vi "MaskThreshold.vi"(7 "fraction":sgl=0.5, 10 "intervals":i32=30, 11 "Mean varS":sgl[][](graph)) -> (2 "Threshold":sgl)   [LabVIEW 2022 SP3]
uses:
  <vilib>/Analysis/NI_AALBase.lvlib
panel:
  out "Waveform Graph":sgl[][](graph)
  out "Histogram Graph":T1(graph)
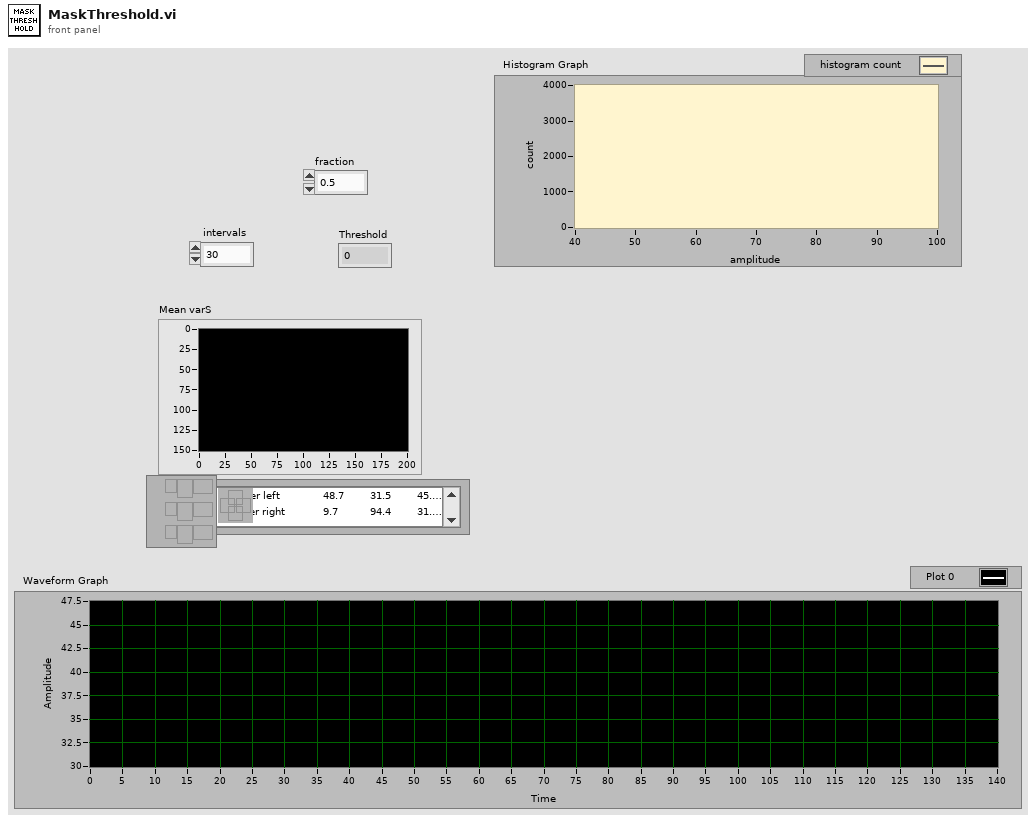
[diagram p1: front panel]
types:
  T1 = cluster{"X Values":dbl[], "Histogram: h(x)":i32[]}
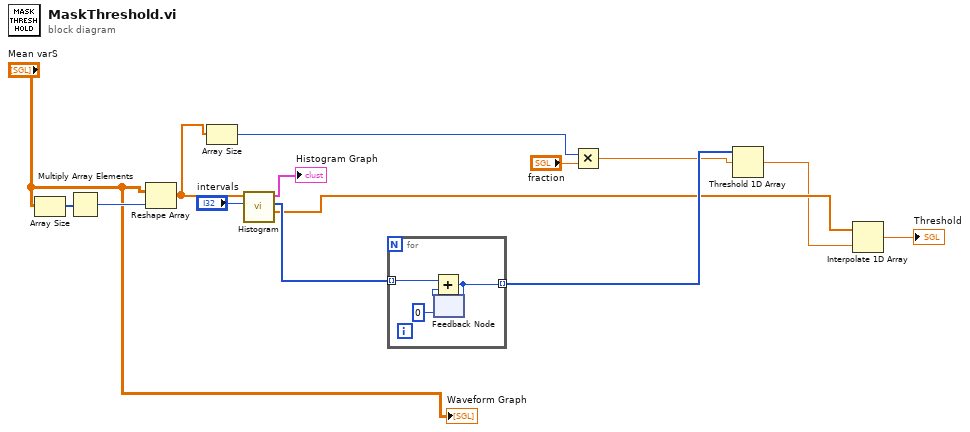
[diagram p0: block diagram]
diagram:
  n1 = Array Size(array="Mean varS") -> (size(s)=w14:i32[])
  n2 = Multiply Array Elements(1:w14) -> (0:w13:i32)
  n3 = Reshape Array("Mean varS", w13) -> (w10:sgl[])
  n4 = Array Size(array=w10) -> (size(s)=w9:i32)
  n5 = call <vilib>:"Histogram.vi"("intervals"="intervals", "X"=w10) -> ("X Values"=w5:dbl[], "Histogram: h(x)"=w6:i32[], "Histogram Graph"=→"Histogram Graph":T1)  [unwired: 6 in, 1 out]
  n6 = for {
    tunnel: w6 -> [w18] mode=indexing
    tunnel: [w16] -> w8 mode=indexing
    n7 = feedback #1(0) -> (w17:i32)
    n8 = Add(x=w18, y=w17) -> (x+y=w16:i32)
    n9 = feedback-in #1(w16) -> ()
  }
  n10 = Multiply(x=w9, y="fraction") -> (x*y=w7:sgl)
  n11 = Threshold 1D Array(2:w7, 3:w8) -> (0:w4:dbl)  [unwired: 1 in]
  n12 = Interpolate 1D Array(1:w4, 2:w5) -> (0:→"Threshold":dbl)
  "Waveform Graph" <- "Mean varS"
